vi "Set Context Menu Item Enabled.vi"(0 "NotifyIcon in":refnum<class "NotifyIcon.lvclass">, 5 "Item Tag":string, 9 "Enabled (True)":bool=TRUE, 11 "error in (no error)":errorcluster) -> (4 "NotifyIcon out":refnum<class "NotifyIcon.lvclass">, 6 "dub Item Tag":string, 15 "error out":errorcluster)   [LabVIEW 2016, in "NotifyIcon.lvclass"]
doc: "Use this VI to enable or disable the MenuItem identified by the <b>Item Tag</b> input. A disabled MenuItem will still display in the Context Menu, but is greyed out and cannot be activated by the user.\n\n\nStinus Olsen\nCIM Industrial Systems A/S\n22. Feb. 2011 15:06\nmailto: seo@cim.as"
uses:
  NotifyIcon.lvclass
panel:
  # "This VI belongs to the NotifyIcon Toolset. \nA toolset that makes it easy to create, control and manipulate a notification icon in the notification area of the Windows taskbar.\nThe toolset requires Microsoft .NET framework 2.0\n\n\nNOTICE -- YOU MUST LEAVE THIS NOTICE IN PLACE.  PER THE TERMS OF THE LICENSE BELOW, YOU MAY SUBLICENSE THIS SOFTWARE \nIN ANY WAY THAT DOES NOT CONFLICT WITH THIS LICENSE.\n\n### BSD License (http://www.opensource.org/licenses/bsd-license.php) Begin ###\n \nCopyright (c) 2011, Stinus Olsen <seo@cim.as>\n\nAll rights reserved.\n\nRedistribution and use in source and binary forms, with or without modification, are permitted provided that the following conditions are met:\n\n    * Redistributions of source code must retain the above copyright notice, this list of conditions and the following disclaimer.\n    * Redistributions in binary form must reproduce the above copyright notice, this list of conditions and the following disclaimer in the \n       documentation and/or other materials provided with the distribution.\n    * Neither the name of CIM Industrial Systems nor the names of its contributors may be used to endorse or promote products derived \n       from this software without specific prior written permission.\n\nTHIS SOFTWARE IS PROVIDED BY THE COPYRIGHT HOLDERS AND CONTRIBUTORS \"AS IS\" AND ANY EXPRESS OR IMPLIED WARRANTIES, \nINCLUDING, BUT NOT LIMITED TO, THE IMPLIED WARRANTIES OF MERCHANTABILITY AND FITNESS FOR A PARTICULAR PURPOSE ARE \nDISCLAIMED. IN NO EVENT SHALL THE COPYRIGHT OWNER OR CONTRIBUTORS BE LIABLE FOR ANY DIRECT, INDIRECT, INCIDENTAL,\n SPECIAL, EXEMPLARY, OR CONSEQUENTIAL DAMAGES (INCLUDING, BUT NOT LIMITED TO, PROCUREMENT OF SUBSTITUTE GOODS OR \nSERVICES; LOSS OF USE, DATA, OR PROFITS; OR BUSINESS INTERRUPTION) HOWEVER CAUSED AND ON ANY THEORY OF LIABILITY, \nWHETHER IN CONTRACT, STRICT LIABILITY, OR TORT (INCLUDING NEGLIGENCE OR OTHERWISE) ARISING IN ANY WAY OUT OF THE USE \nOF THIS SOFTWARE, EVEN IF ADVISED OF THE POSSIBILITY OF SUCH DAMAGE.\n\n### BSD License End ###"
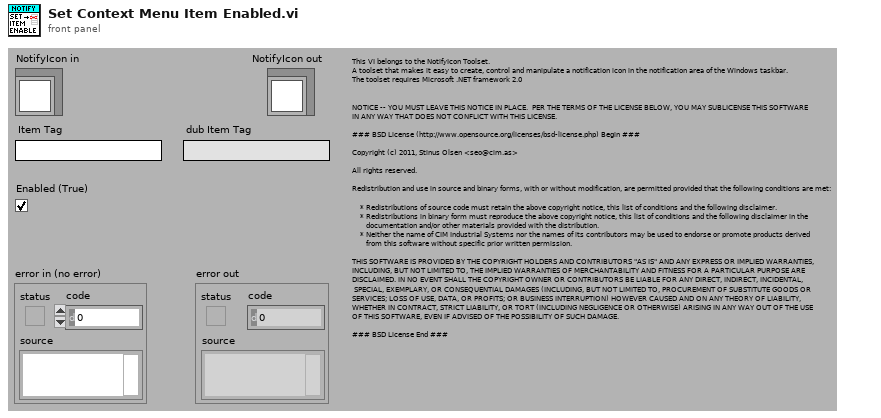
[diagram p1: front panel]
types:
  T1 = typedef "NotifyIcon.lvclass/MenuItem Properties.ctl" = cluster{"Enabled":bool, "Visible":bool, "DefaultItem":bool, "Checked":bool, "RadioCheck":bool, "Break":bool, "BarBreak":bool, "Text":string}
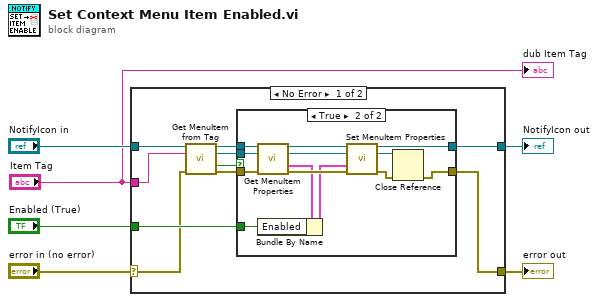
[diagram p0: block diagram]
diagram:
  n1 = case shown="No Error" "error in (no error)" {
    selector: "error in (no error)" -> [w8 w33]
    tunnel: [w7 w33] -> w5
    tunnel: [w10 w32] -> w3
    tunnel: "NotifyIcon in" -> [w15 w32]
    tunnel: "Item Tag" -> [w16 _]
    tunnel: "Enabled (True)" -> [w9 _]
    frame No Error {
      n2 = call "Get MenuItem from Tag.vi"("NotifyIcon in"=w15, "Item Tag"=w16, "error in (no error)"=w8) -> ("NotifyIcon out"=w14:refnum<class "NotifyIcon.lvclass">, "MenuItem"=w11:refnum<k24>, "Found"=w13:bool, "error out"=w12:errorcluster)  [unwired: 9 out]
      n3 = case shown="True" w13 {
        tunnel: w14 -> [w18 w31]
        tunnel: w12 -> [w17 w29]
        tunnel: w11 -> [_ w30]
        tunnel: [w18 w25] -> w10
        tunnel: w9 -> [_ w23]
        tunnel: [w17 w19] -> w7
        frame False {
        }
        frame True {
          n4 = call "Get MenuItem Properties.vi"("NotifyIcon in"=w31, "MenuItem"=w30, "error in (no error)"=w29) -> ("dub NotifyIcon"=w28:refnum<class "NotifyIcon.lvclass">, "MenuItem out"=w27:refnum<k24>, "MenuItem Properties"=w24:T1, "error out"=w26:errorcluster)  [unwired: 9 out]
          n5 = Bundle By Name(cluster=w24, "Enabled"=w23) -> (w22:T1)
          n6 = call "Set MenuItem Properties.vi"("NotifyIcon in"=w28, "MenuItem"=w27, "MenuItem Properties"=w22, "error in (no error)"=w26) -> ("dub NotifyIcon"=w25:refnum<class "NotifyIcon.lvclass">, "MenuItem out"=w21:refnum<k24>, "error out"=w20:errorcluster)  [unwired: 9 out]
          n7 = Close Reference(reference=w21, error in (no error)=w20) -> (error out=w19:errorcluster)
        }
      }
    }
    frame Error {
    }
  }
  "error out" <- w5
  "NotifyIcon out" <- w3
  "dub Item Tag" <- "Item Tag"
